vi "Define Mask.vi"(8 "error in (no error)":errorcluster, 11 "FPGA Image":T2(plugin-control)=refnum) -> (0 "error out":errorcluster)   [LabVIEW 2013]
doc: "GUI for selecting a part type and starting a batch process\nPart types list is passed in from caller.\nReturns when Start or Cancel is pressed."
uses:
  Sectors/Number of Wing Sector.ctl
  Mask ROI FG Enum.ctl
  Mask ROI Cluster.ctl
  Common/File IO/INI/Read write mode.ctl
  Message Passing/MsgQ Loops enum.ctl
  Common/State Machines/State Machine Lib.lvlib
  Common/GUI/GUI.lvlib
  <vilib>/vision/NI_Vision_Development_Module.lvlib
  Image Processing.lvlib
  Message Passing/Main MsgQ.lvlib
panel:
  out "[Avg BG]":dbl[](array[numeric])
  in  "NumWingSectors":T1=1 items=["1"=1, "2"=2, "4"=4, "8"=8, "16"=16]
  out "State":string
  in  "Exit":bool
  in  "Save Mask":bool
  out "combo mask":T2(plugin-control)
  out "right mask":T2(plugin-control)
  out "right masked image":T2(plugin-control)
  out "right annulus":T3={"Center X"=929, "Center Y"=663, "Inner Radius"=200, "Outer Radius"=405, "Start Angle"=90.0, "End Angle"=180.0} {"End Angle" format="%.2f"; "Start Angle" format="%.2f"; "Center X" scale=0.0..1024.0}
  out "left mask":T2(plugin-control)
  out "left masked image":T2(plugin-control)
  out "left annulus":T3={"Center X"=929, "Center Y"=663, "Inner Radius"=200, "Outer Radius"=405, "Start Angle"=90.0, "End Angle"=180.0} {"End Angle" format="%.2f"; "Start Angle" format="%.2f"; "Center X" scale=0.0..1024.0}
  in  "Accept Threshold":bool
  out "Processed Image":T2(plugin-control)
  in  "Threshold Range":cluster{"Lower value":dbl, "Upper value":dbl}={"Lower value"=106.82432432432432, "Upper value"=255.0} {"Upper value" min=0.0 max=255.0 scale=0.0..255.0; "Lower value" min=0.0 max=255.0 scale=0.0..255.0}
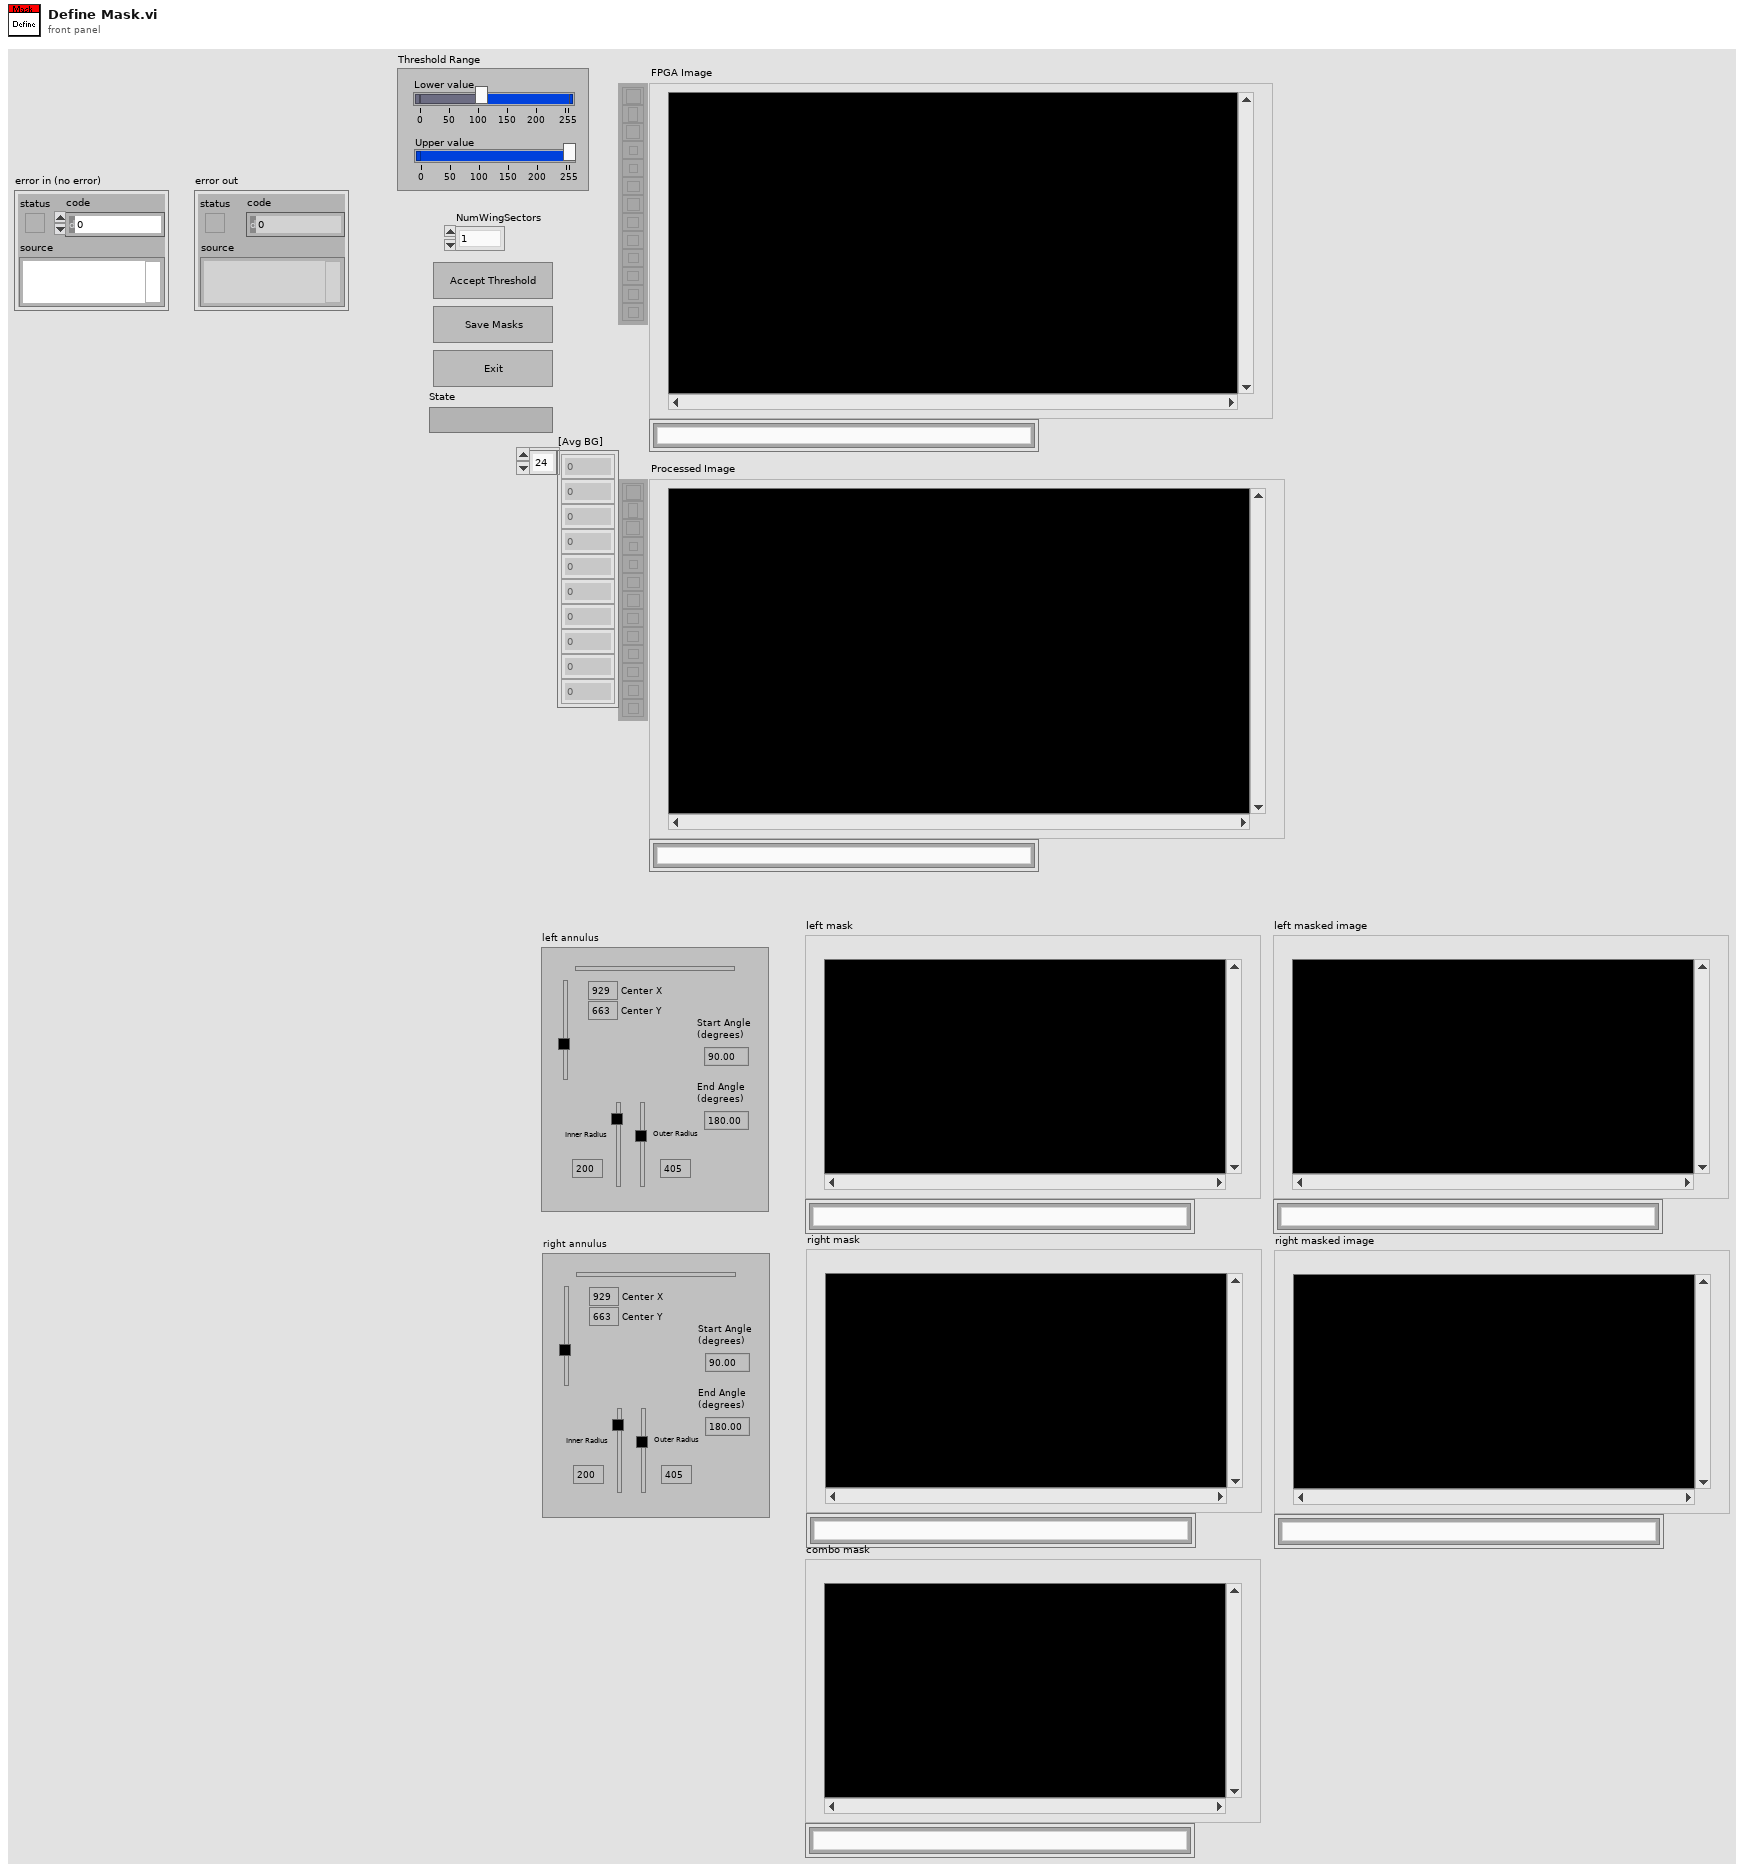
[diagram p1: front panel]
types:
  T1 = typedef "Number of Wing Sector.ctl" = u8
  T2 = typedef "IMAQ Image.ctl" = refnum<image>
  T3 = typedef "IMAQ Circle" = cluster{"Center X":i32, "Center Y":i32, "Inner Radius":i32, "Outer Radius":i32, "Start Angle":dbl, "End Angle":dbl}
  T4 = typedef "State Machine Lib.lvlib/STATE cluster.ctl" = cluster{"State":string, "Parameters":variant}
  T5 = typedef "Mask ROI FG Enum.ctl" = enum16{"Read", "Write"}
  T6 = typedef "Main MsgQ.lvlib/MsgQ Loops enum.ctl" = enum16{"User Interface", "Image Acq"}
  T7 = typedef "Read write mode.ctl" = enum16{"Read", "Write"}
  T8 = typedef "Mask ROI Cluster.ctl" = cluster{"left annulus":T3, "right annulus":T3, "Threshold Range":cluster{"Lower value":dbl, "Upper value":dbl}, "[Avg BG]":u8[], "Number of Sectors":u8}
  T9 = typedef "Sector Parameter Cluster.ctl" = cluster{"Start Angle":fxp<+,17,3>, "End Angle":fxp<+,17,3>, "Inner Radius":u16, "Outter Radius":u16, "Hinge X":u16, "Hinge Y":u16, "NumWingSectors":u8}
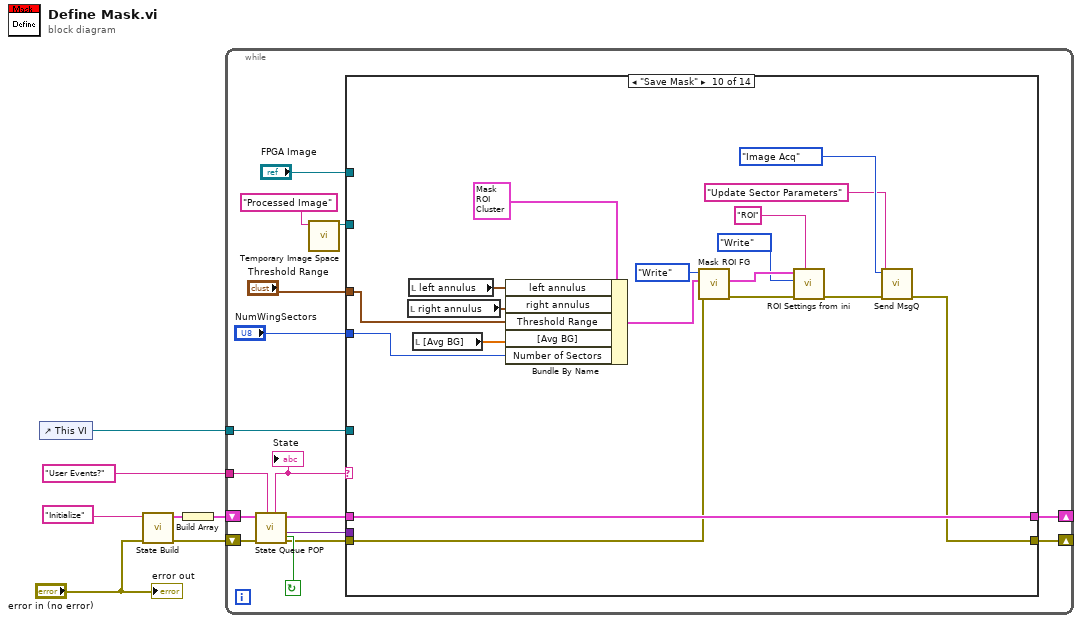
[diagram p0: block diagram]
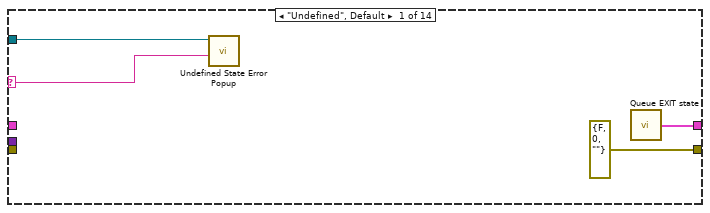
[diagram p2: hidden frame]
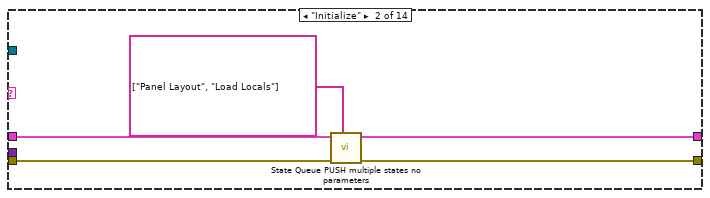
[diagram p3: hidden frame]
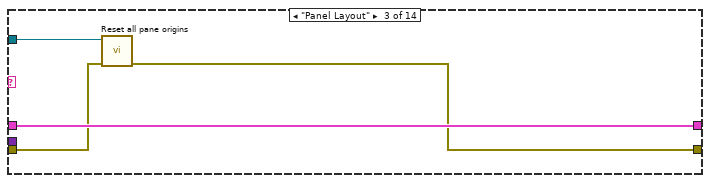
[diagram p4: hidden frame]
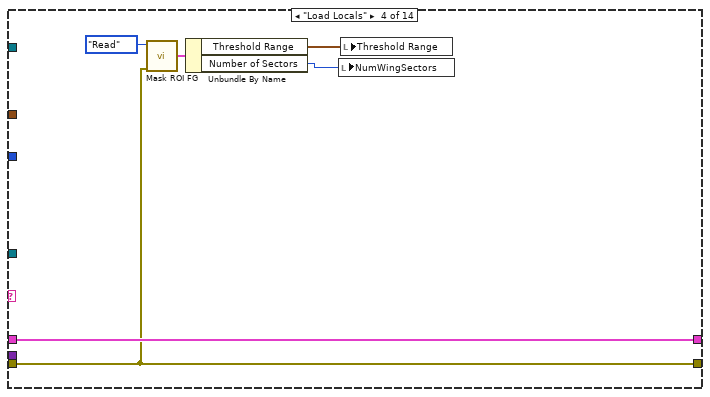
[diagram p5: hidden frame]
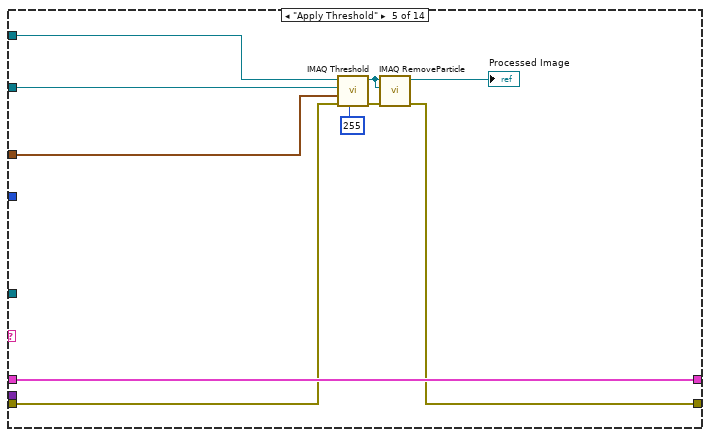
[diagram p6: hidden frame]
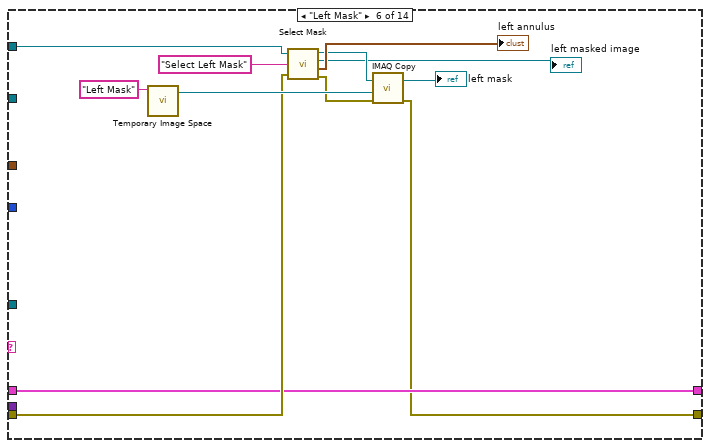
[diagram p7: hidden frame]
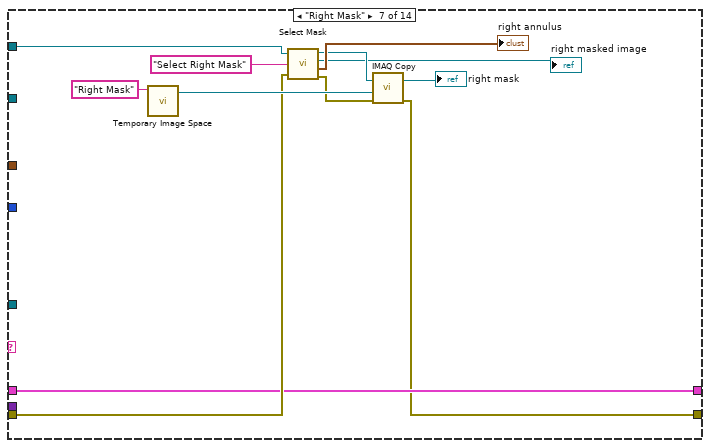
[diagram p8: hidden frame]
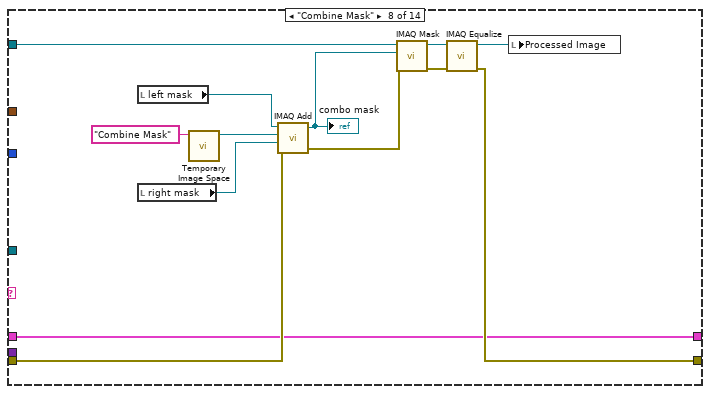
[diagram p9: hidden frame]
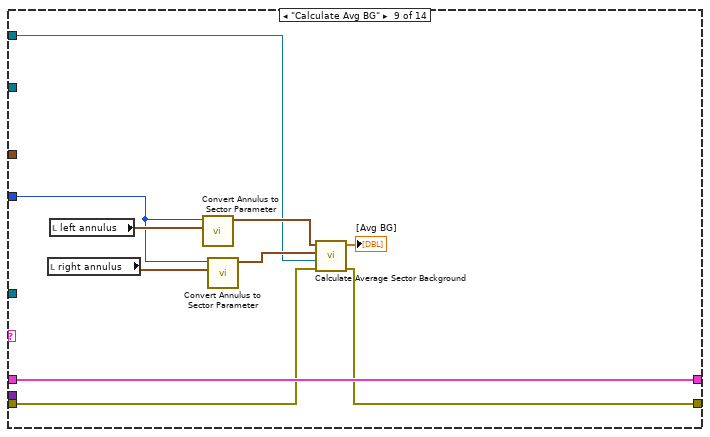
[diagram p10: hidden frame]
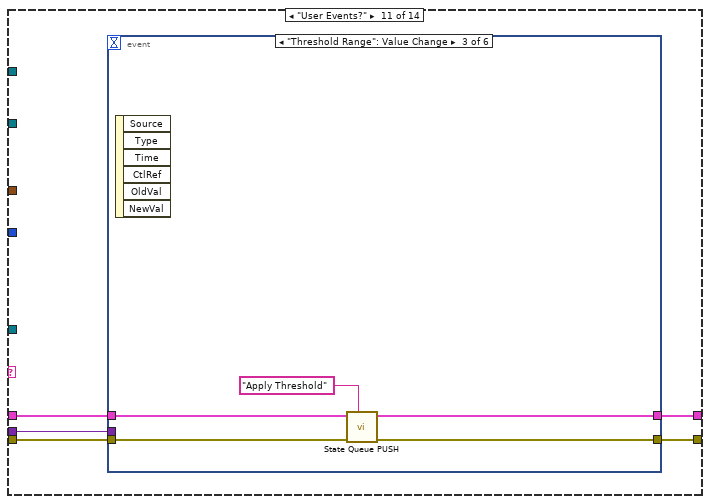
[diagram p11: hidden frame]
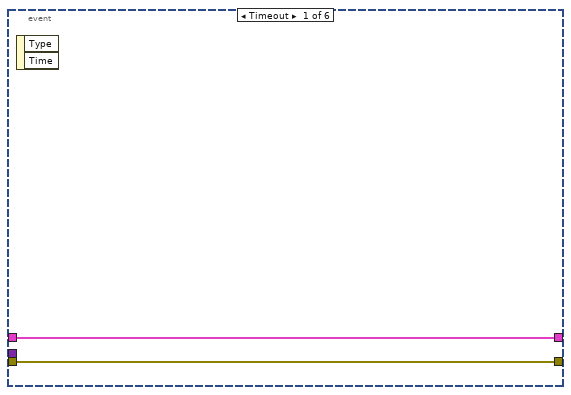
[diagram p12: hidden frame]
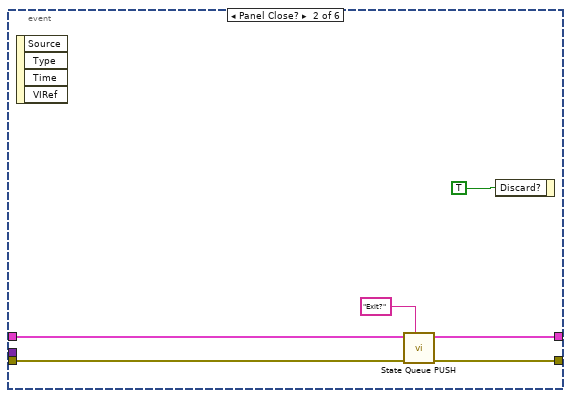
[diagram p13: hidden frame]
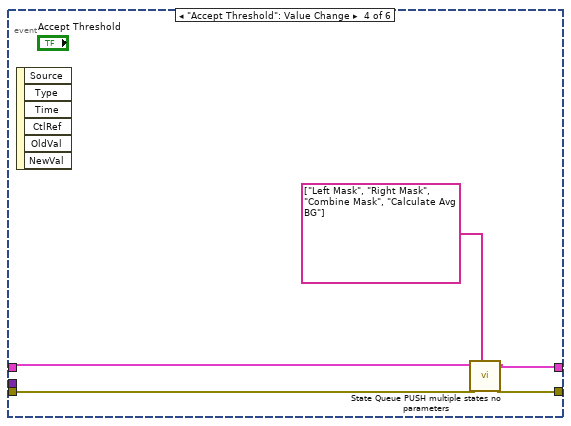
[diagram p14: hidden frame]
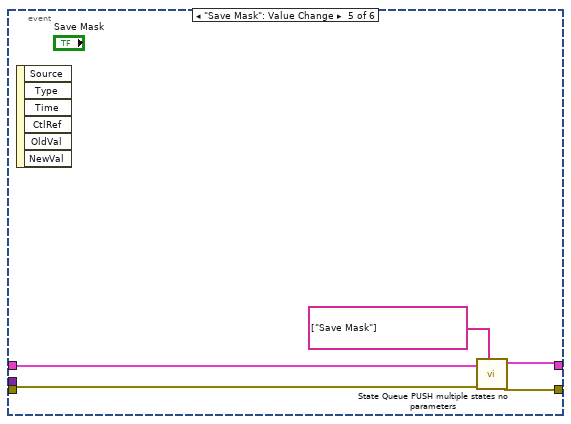
[diagram p15: hidden frame]
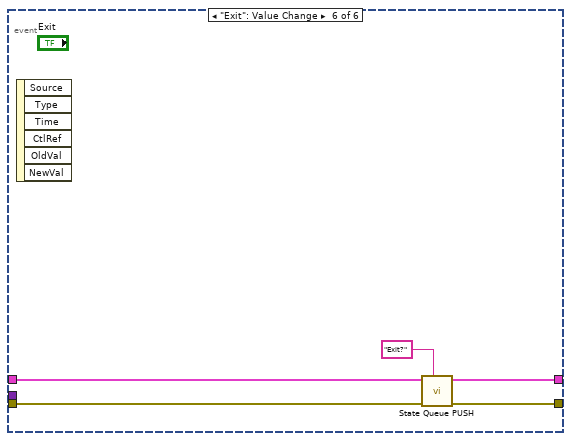
[diagram p16: hidden frame]
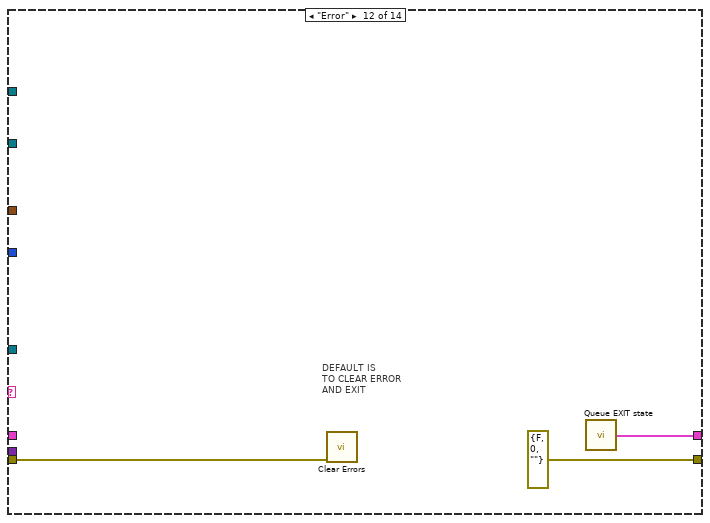
[diagram p17: hidden frame]
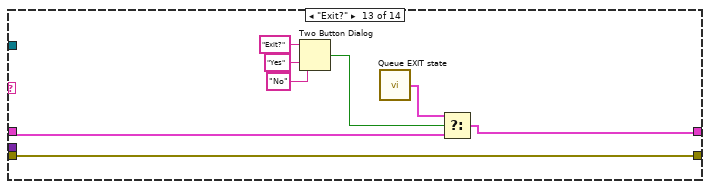
[diagram p18: hidden frame]
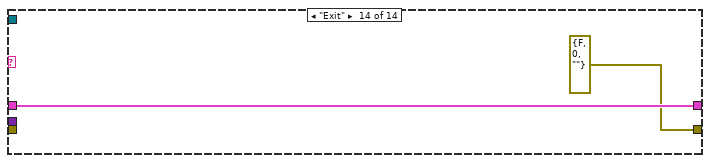
[diagram p19: hidden frame]
diagram:
  n1 = control-ref of="This VI"() -> (w6:refnum<vi>)
  n2 = call "State Build.vi"("error in (no error)"="error in (no error)", "State"="Initialize") -> ("error out"=w3:errorcluster, "State Out"=w4:T4)  [unwired: 8 in]
  n3 = Build Array(w4) -> (w5:T4[])
  n4 = while {
    shift-right: [w14] -> _
    shift-left: w3 -> [w22]
    shift-right: [w13] -> _
    shift-left: w5 -> [w20]
    tunnel: "User Events?" ("Default state") -> [w21]
    tunnel: w6 -> [w16]
    stop <- w23 continue-if-true
    n5 = call "State Queue POP.vi"("Default state"=w21, "error in (no error)"=w22, "State que in"=w20) -> ("error out"=w19:errorcluster, "Parameters"=w15:variant, "State que out"=w18:T4[], "Not Exit?"=w23:bool, "State case out"=w17:string)  [unwired: 4 out]
    "State" <- w17
    n6 = call "Temporary Image Space.vi"("Image Name"="Processed Image") -> ("Image Out"=w10:T2)  [unwired: 10 in]
    n7 = case shown="\"Save Mask\"" w17 {
      selector: w17 -> [w24 _ _ _ _ _ _ _ _ _ _ _ _ _]
      tunnel: w19 -> [_ w30 w34 w41 w47 w56 w68 w82 w98 w110 w121 w151 w161 _]
      tunnel: w18 -> [_ w32 w36 w42 w48 w55 w67 w77 w99 w117 w122 _ w155 w163]
      tunnel: w16 -> [w25 _ w35 _ _ _ _ _ _ _ _ _ _ _]
      tunnel: w15 -> [_ _ _ _ _ _ _ _ _ _ w120 _ _ _]
      tunnel: [errorcluster {"status"=FALSE, "code"=0, "source"=""} ("error out") w31 w33 w41 w46 w54 w66 w78 w97 w100 w119 errorcluster {"status"=FALSE, "code"=0, "source"=""} ("error out") w161 errorcluster {"status"=FALSE, "code"=0, "source"=""} ("error out")] -> w14
      tunnel: [w27 w28 w36 w42 w48 w55 w67 w77 w99 w117 w118 w152 w154 w163] -> w13
      tunnel: "Threshold Range" -> [_ _ _ _ w45 _ _ _ _ w112 _ _ _ _]
      tunnel: "FPGA Image" -> [_ _ _ _ w44 w57 w69 _ w92 _ _ _ _ _]
      tunnel: w10 -> [_ _ _ _ w43 _ _ w81 _ _ _ _ _ _]
      tunnel: "NumWingSectors" -> [_ _ _ _ _ _ _ _ w90 w108 _ _ _ _]
      frame "Undefined", Default {
        n8 = call "Undefined State Error Popup.vi"("String"=w24, "This VI (Caller if unwired)"=w25) -> ()  [unwired: 10 out]
        n9 = call "Queue EXIT state.vi"() -> ("Exit State Q"=w27:T4[])  [unwired: 1 in]
      }
      frame "Initialize" {
        n10 = call "State Queue PUSH multiple states no parameters.vi"("States to queue"=string[] ["Panel Layout", "Load Locals"], "error in (no error)"=w30, "State que in"=w32) -> ("error out"=w31:errorcluster, "State que out"=w28:T4[])  [unwired: 1 in, 6 out]
      }
      frame "Panel Layout" {
        n11 = call "Reset all pane origins.vi"("error in (no error"=w34, "Vi Ref In"=w35) -> ("error out"=w33:errorcluster)  [unwired: 9 out]
      }
      frame "Load Locals" {
        n12 = call "Mask ROI FG.vi"("error in (no error)"=w41, "Operation"=Mask_ROI_FG_Enum."Read") -> ("Mask ROI Out"=w39:T8)  [unwired: 8 in, 1 out]
        n13 = Unbundle By Name(w39) -> ("Threshold Range"=w38:cluster{"Lower value":dbl, "Upper value":dbl}, "Number of Sectors"=w37:u8)
        n14 = local write "NumWingSectors"(w37) -> ()
        n15 = local write "Threshold Range"(w38) -> ()
      }
      frame "Apply Threshold" {
        n16 = call "IMAQ Threshold"("Replace Value"=u8 255, "error in (no error)"=w47, "Range"=w45, "Image Dst"=w43, "Image Src"=w44) -> ("error out"=w50:errorcluster, "Image Dst Out"=w52:T2)  [unwired: 1 in, 4 out]
        n17 = call "IMAQ RemoveParticle"("error in (no error)"=w50, "Image Dst"=w52, "Image Src"=w52) -> ("error out"=w46:errorcluster, "Image Dst Out"=→"Processed Image":T2)  [unwired: 4 in, 3 out]
      }
      frame "Left Mask" {
        n18 = call "Temporary Image Space.vi"("Image Name"="Left Mask") -> ("Image Out"=w58:T2)  [unwired: 10 in]
        n19 = call "Select Mask.vi"("Read \nImage"=w57, "Prompt"="Select Left Mask", "error in"=w56) -> ("mask"=w61:T2, "Masked \nImage"=→"left masked image":T2, "Annulus"=→"left annulus":T3, "error out"=w53:errorcluster)  [unwired: 1 out]
        n20 = call "IMAQ Copy"("error in (no error)"=w53, "Image Dst"=w58, "Image Src"=w61) -> ("error out"=w54:errorcluster, "Image Dst Out"=→"left mask":T2)  [unwired: 3 in]
      }
      frame "Right Mask" {
        n21 = call "Temporary Image Space.vi"("Image Name"="Right Mask") -> ("Image Out"=w70:T2)  [unwired: 10 in]
        n22 = call "Select Mask.vi"("Read \nImage"=w69, "Prompt"="Select Right Mask", "error in"=w68) -> ("mask"=w73:T2, "Masked \nImage"=→"right masked image":T2, "Annulus"=→"right annulus":T3, "error out"=w65:errorcluster)  [unwired: 1 out]
        n23 = call "IMAQ Copy"("error in (no error)"=w65, "Image Dst"=w70, "Image Src"=w73) -> ("error out"=w66:errorcluster, "Image Dst Out"=→"right mask":T2)  [unwired: 3 in]
      }
      frame "Combine Mask" {
        n24 = local read "left mask"() -> (w84:T2)
        n25 = local read "right mask"() -> (w83:T2)
        n26 = call "Temporary Image Space.vi"("Image Name"="Combine Mask") -> ("Image Out"=w86:T2)  [unwired: 10 in]
        n27 = call "IMAQ Add"("Image Src A"=w84, "Image Dst"=w86, "Image Src B"=w83, "error in (no error)"=w82) -> ("Image Dst Out"=w87:T2, "error out"=w79:errorcluster)  [unwired: 3 in]
        "combo mask" <- w87
        n28 = call "IMAQ Mask"("error in (no error)"=w79, "Image Mask"=w87, "Image Src"=w81) -> ("error out"=w88:errorcluster, "Image Dst Out"=w89:T2)  [unwired: 1 in, 1 out]
        n29 = call "IMAQ Equalize"("error in (no error)"=w88, "Image Src"=w89) -> ("error out"=w78:errorcluster, "Image Dst Out"=w80:T2)  [unwired: 4 in, 4 out]
        n30 = local write "Processed Image"(w80) -> ()
      }
      frame "Calculate Avg BG" {
        n31 = local read "right annulus"() -> (w95:T3)
        n32 = local read "left annulus"() -> (w96:T3)
        n33 = call "Convert Annulus to Sector Parameter.vi"("Annulus"=w96, "NumWingSectors"=w90) -> ("Sector Parameter"=w94:T9)  [unwired: 9 in]
        n34 = call "Convert Annulus to Sector Parameter.vi"("Annulus"=w95, "NumWingSectors"=w90) -> ("Sector Parameter"=w93:T9)  [unwired: 9 in]
        n35 = call "Calculate Average Sector Background.vi"("error in (no error)"=w98, "Image"=w92, "Right Sector Parameters"=w93, "Left Sector Parameters"=w94) -> ("error out"=w97:errorcluster, "[Avg BG]"=→"[Avg BG]":dbl[])  [unwired: 6 in]
      }
      frame "Save Mask" {
        n36 = local read "right annulus"() -> (w114:T3)
        n37 = local read "left annulus"() -> (w113:T3)
        n38 = local read "[Avg BG]"() -> (w109:dbl[])
        n39 = Bundle By Name(cluster=T8 {"left annulus"={"Center X"=929, "Center Y"=663, "Inner Radius"=200, "Outer Radius"=405, "Start Angle"=90.0, "End Angle"=180.0}, "right annulus"={"Center X"=929, "Center Y"=663, "Inner Radius"=200, "Outer Radius"=405, "Start Angle"=90.0, "End Angle"=180.0}, "Threshold Range"={"Lower value"=106.82432432432432, "Upper value"=255.0}, "[Avg BG]"=[], "Number of Sectors"=0} ("Mask ROI In"), "left annulus"=w113, "right annulus"=w114, "Threshold Range"=w112, "[Avg BG]"=w109, "Number of Sectors"=w108) -> (w111:T8)
        n40 = call "Mask ROI FG.vi"("error in (no error)"=w110, "Mask ROI In"=w111, "Operation"=Mask_ROI_FG_Enum."Write") -> ("error out"=w105:errorcluster, "Mask ROI Out"=w107:T8)  [unwired: 7 in]
        n41 = call "ROI Settings from ini.vi"("Section"="ROI", "error in (no error)"=w105, "Operation"=Read_write_mode."Write", "Mask ROI In"=w107) -> ("error out"=w101:errorcluster)  [unwired: 5 in, 2 out]
        n42 = call "Send MsgQ.vi"("error in (no error)"=w101, "Message String"="Update Sector Parameters", "Send to MsgQ"=MsgQ_Loops_enum."Image Acq") -> ("error out"=w100:errorcluster)  [unwired: 8 in]
      }
      frame "User Events?" {
        n43 = event shown="[2] \"Threshold Range\": Value Change" {
          selector: _ -> [_ _ _ _ _ _]
          dyn-events: _ -> [_ _ _ _ _ _]
          timeout: _ -> [_ _ _ _ _ _]
          tunnel: w122 -> [w123 w129 w135 w138 w144 w147]
          tunnel: w121 -> [w124 w128 w134 w136 w141 w148]
          tunnel: w120 -> [_ _ _ _ _ _]
          tunnel: [w124 w126 w132 w139 w142 w149] -> w119
          tunnel: [w123 w127 w133 w140 w143 w150] -> w118
          event Timeout {
            n44 = event-data() -> ()  [unwired: 3 out]
          }
          event Panel Close? {
            n45 = event-data() -> ()  [unwired: 5 out]
            n46 = call "State Queue PUSH.vi"("State case"="Exit?", "error in (no error)"=w128, "State que in"=w129) -> ("error out"=w126:errorcluster, "State que out"=w127:T4[])  [unwired: 2 in, 5 out]
            n47 = event-data("Discard?"=TRUE) -> ()  [unwired: 1 in, 1 out]
          }
          event "Threshold Range": Value Change {
            n48 = event-data() -> ()  [unwired: 7 out]
            n49 = call "State Queue PUSH.vi"("State case"="Apply Threshold", "error in (no error)"=w134, "State que in"=w135) -> ("error out"=w132:errorcluster, "State que out"=w133:T4[])  [unwired: 2 in, 5 out]
          }
          event "Accept Threshold": Value Change {
            n50 = event-data() -> ()  [unwired: 7 out]
            n51 = call "State Queue PUSH multiple states no parameters.vi"("States to queue"=string[] ["Left Mask", "Right Mask", "Combine Mask", "Calculate Avg BG"], "error in (no error)"=w136, "State que in"=w138) -> ("error out"=w139:errorcluster, "State que out"=w140:T4[])  [unwired: 7 in]
          }
          event "Save Mask": Value Change {
            n52 = event-data() -> ()  [unwired: 7 out]
            n53 = call "State Queue PUSH multiple states no parameters.vi"("States to queue"=string[] ["Save Mask"], "error in (no error)"=w141, "State que in"=w144) -> ("error out"=w142:errorcluster, "State que out"=w143:T4[])  [unwired: 7 in]
          }
          event "Exit": Value Change {
            n54 = event-data() -> ()  [unwired: 7 out]
            n55 = call "State Queue PUSH.vi"("State case"="Exit?", "error in (no error)"=w148, "State que in"=w147) -> ("error out"=w149:errorcluster, "State que out"=w150:T4[])  [unwired: 7 in]
          }
        }
      }
      frame "Error" {
        # "DEFAULT IS \nTO CLEAR ERROR\nAND EXIT"
        n56 = call <vilib>:"Clear Errors.vi"("error in (no error)"=w151) -> ()  [unwired: 7 out]
        n57 = call "Queue EXIT state.vi"() -> ("Exit State Q"=w152:T4[])  [unwired: 1 in]
      }
      frame "Exit?" {
        n58 = Two Button Dialog(message="Exit?", 1:"No" ("F button name (\"Cancel\")"), 2:"Yes" ("T button name (\"OK\")")) -> (T button?=w157:bool)
        n59 = call "Queue EXIT state.vi"() -> ("Exit State Q"=w156:T4[])  [unwired: 1 in]
        n60 = Select(t=w156, s=w157, f=w155) -> (s? t:f=w154:T4[])
      }
      frame "Exit" {
      }
    }
  }
  "error out" <- "error in (no error)"
